vi "Save_Load_Graph_Setup.vi"(3 "Setup String in":string, 4 "Graph Number":i32=1 min=1 max=10, 5 "Mode":T3(ring), 6 "Graph in":T2={"Plot 1"=1, "Plot 2"=3, "Save graph"=0, "Plot Type"=enum."Voltage trace"} {"Save graph" items=["Do not save plot", "Save plot"]; "Plot 2" items=["Nothing", "Velocity1", "Arr time1", "Velocity2", "Arr time2"]; "Plot 1" items=["Nothing", "Velocity1", "Arr time1", "Velocity2", "Arr time2"]}) -> (0 "Setup String Out":string, 1 "Variables found?":bool, 2 "Graph Out":T2={"Plot 1"=1, "Plot 2"=3, "Save graph"=0, "Plot Type"=enum."Voltage trace"} {"Save graph" items=["Do not save plot", "Save plot"]; "Plot 2" items=["Nothing", "Velocity1", "Arr time1", "Velocity2", "Arr time2"]; "Plot 1" items=["Nothing", "Velocity1", "Arr time1", "Velocity2", "Arr time2"]})   [LabVIEW 2020]
uses:
  Controls/Graph_Type.ctl
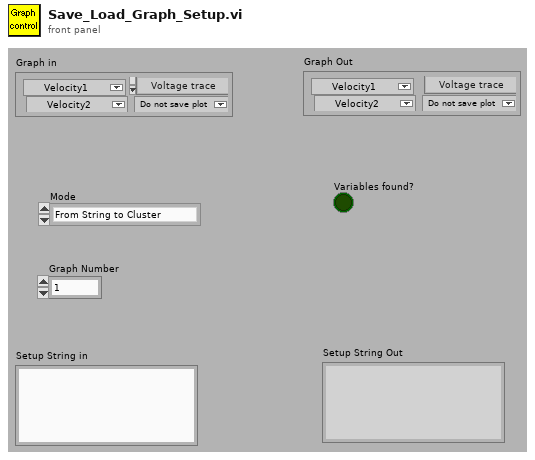
[diagram p1: front panel]
types:
  T1 = typedef "Graph_Type.ctl" = enum16{"Show no graph", "Voltage trace", "Velocity trace", "Vel histogram", "Spectrum", "f.E(f) v Log f", "Auto-Corr"}
  T2 = cluster{"Plot 1":u16, "Plot 2":u16, "Save graph":u16, "Plot Type":T1}
  T3 = enum16{"From String to Cluster", "From Cluster to String"}
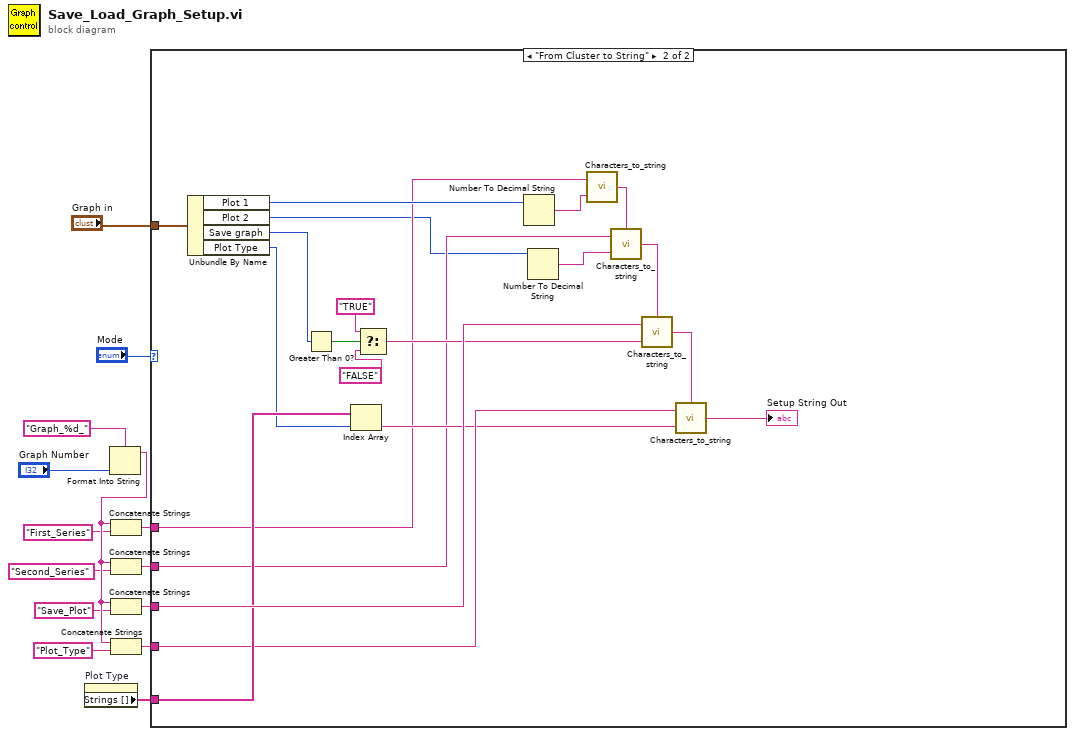
[diagram p0: block diagram]
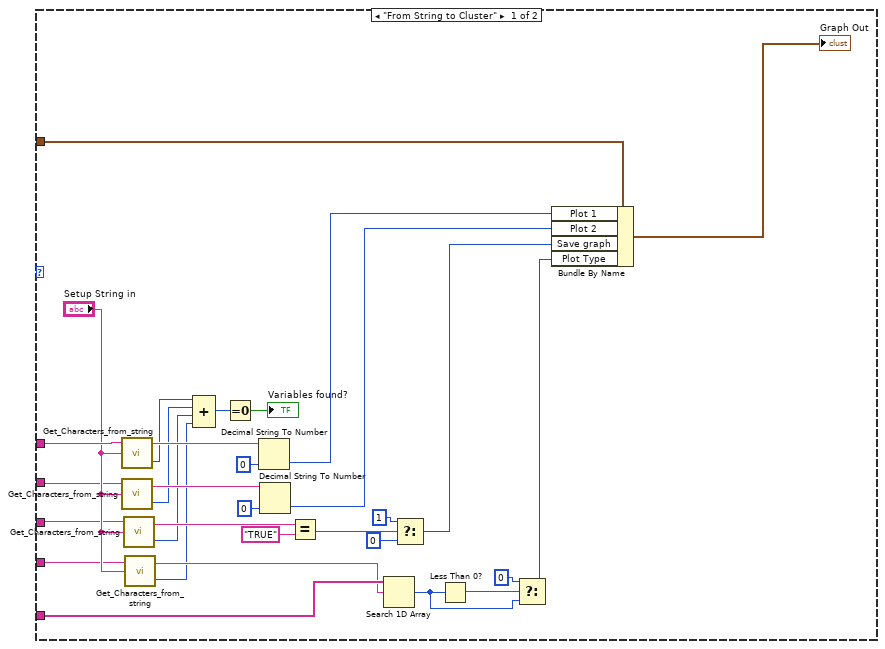
[diagram p2: hidden frame]
diagram:
  n1 = property on="Plot Type" class="Enum (strict)"() -> ("Strings []"=w2:string[])  [unwired: 2 in, 2 out]
  n2 = Format Into String(format string="Graph_%d_", "Graph Number") -> (resulting string=w10:string)  [unwired: 2 in, 1 out]
  n3 = Concatenate Strings(w10, "First_Series") -> (w5:string)
  n4 = Concatenate Strings(w10, "Second_Series") -> (w4:string)
  n5 = Concatenate Strings(w10, "Save_Plot") -> (w3:string)
  n6 = Concatenate Strings(w10, "Plot_Type") -> (w1:string)
  n7 = case shown="\"From Cluster to String\"" "Mode" {
    tunnel: "Graph in" -> [w45 w66]
    tunnel: w5 -> [w43 w54]
    tunnel: w4 -> [w41 w53]
    tunnel: w3 -> [w40 w63]
    tunnel: w2 -> [w26 w59]
    tunnel: w1 -> [w39 w58]
    frame "From String to Cluster" {
      n8 = call "Get_Characters_from_string.vi"("Input string"="Setup String in", "Variable name"=w43) -> ("Status"=w17:enum16{"Char in string", "Char not in string"}, "Value"=w38:string)  [unwired: 1 in]
      n9 = call "Get_Characters_from_string.vi"("Input string"="Setup String in", "Variable name"=w41) -> ("Status"=w18:enum16{"Char in string", "Char not in string"}, "Value"=w36:string)  [unwired: 1 in]
      n10 = call "Get_Characters_from_string.vi"("Input string"="Setup String in", "Variable name"=w40) -> ("Status"=w19:enum16{"Char in string", "Char not in string"}, "Value"=w32:string)  [unwired: 1 in]
      n11 = call "Get_Characters_from_string.vi"("Input string"="Setup String in", "Variable name"=w39) -> ("Status"=w20:enum16{"Char in string", "Char not in string"}, "Value"=w25:string)  [unwired: 1 in]
      n12 = Compound Arithmetic op=unknown(w17, w18, w19, w20) -> (w16:u16)
      n13 = Equal To 0?(x=w16) -> (x = 0?=→"Variables found?":bool)
      n14 = Decimal String To Number(string=w38, default (0L)=0 ("default (0 I32)")) -> (number=w37:i32)  [unwired: 2 out]
      n15 = Decimal String To Number(string=w36, default (0L)=0 ("default (0 I32)")) -> (number=w35:i32)  [unwired: 2 out]
      n16 = Equal?(x=w32, y="TRUE") -> (x = y?=w30:bool)
      n17 = Search 1D Array(1D array=w26, element=w25) -> (index of element=w22:i32)  [unwired: 1 out]
      n18 = Select(t=1, s=w30, f=0) -> (s? t:f=w27:i32)
      n19 = Less Than 0?(x=w22) -> (x < 0?=w24:bool)
      n20 = Select(t=0, s=w24, f=w22) -> (s? t:f=w23:i32)
      n21 = Bundle By Name(cluster=w45, "Plot 1"=w37, "Plot 2"=w35, "Save graph"=w27, "Plot Type"=w23) -> (→"Graph Out":T2)
    }
    frame "From Cluster to String" {
      n22 = Unbundle By Name(w66) -> ("Plot 1"=w55:u16, "Plot 2"=w51:u16, "Save graph"=w65:u16, "Plot Type"=w56:T1)
      n23 = Greater Than 0?(x=w65) -> (x > 0?=w64:bool)
      n24 = Index Array(array=w59, index=w56) -> (element=w57:string)
      n25 = Select(t="TRUE", s=w64, f="FALSE") -> (s? t:f=w62:string)
      n26 = Number To Decimal String(number=w55) -> (decimal integer string=w52:string)  [unwired: 1 out]
      n27 = Number To Decimal String(number=w51) -> (decimal integer string=w50:string)  [unwired: 1 out]
      n28 = call "Characters_to_string.vi"("Characters to write"=w52, "Label for characters"=w54) -> ("Output string"=w47:string)  [unwired: 1 in]
      n29 = call "Characters_to_string.vi"("stringIn"=w47, "Characters to write"=w50, "Label for characters"=w53) -> ("Output string"=w48:string)
      n30 = call "Characters_to_string.vi"("stringIn"=w48, "Characters to write"=w62, "Label for characters"=w63) -> ("Output string"=w49:string)
      n31 = call "Characters_to_string.vi"("stringIn"=w49, "Characters to write"=w57, "Label for characters"=w58) -> ("Output string"=→"Setup String Out":string)
    }
  }
